vi "Corr Transducers Get Unity Corrections.vi"() -> (1 "dummy.vd path":path, 2 "dummy.cs path":path)   [LabVIEW 2020]
doc: "Returns unity corrections for CS and VD from the project example transducers corrections folder."
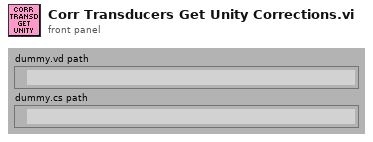
[diagram p1: front panel]
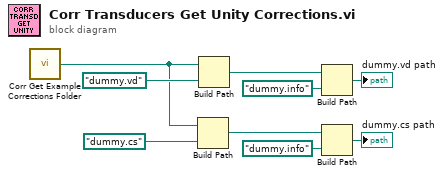
[diagram p0: block diagram]
diagram:
  n1 = call "Corr Get Example Corrections Folder.vi"() -> ("transducers path"=w7:path)  [unwired: 1 in, 2 out]
  n2 = Build Path(base path=w7, name or relative path=path "dummy.cs") -> (appended path=w3:path)
  n3 = Build Path(base path=w7, name or relative path=path "dummy.vd") -> (appended path=w6:path)
  n4 = Build Path(base path=w6, name or relative path=path "dummy.info") -> (appended path=→"dummy.vd path":path)
  n5 = Build Path(base path=w3, name or relative path=path "dummy.info") -> (appended path=→"dummy.cs path":path)
